vi "element_editor_hydroyse_run.vi"(10 "Break":refnum<vi>) -> ()   [LabVIEW 2019]
uses:
  lib/libSimulationControl/libSimulationControl.lvlib
panel:
  out "spec":path
  # "*******************************************************************\nBiogas Plant Control\n\nAuthor: Paul Zügel\nGCSC-Frankfurt am Main 2020\n\n*******************************************************************"
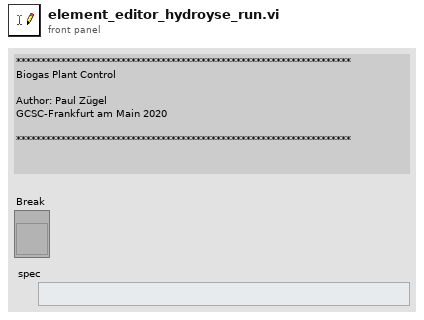
[diagram p1: front panel]
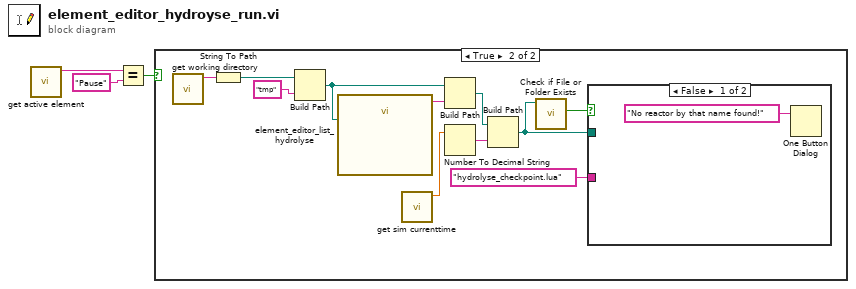
[diagram p0: block diagram]
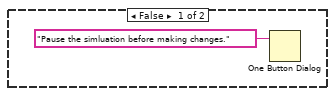
[diagram p2: hidden frame]
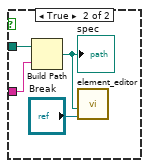
[diagram p3: hidden frame]
diagram:
  n1 = call "get active element.vi"() -> ("active_element"=w3:string)  [unwired: 10 in, 1 out]
  n2 = Equal?(x=w3, y="Pause") -> (x = y?=w1:bool)
  n3 = case shown="True" w1 {
    frame False {
      n4 = One Button Dialog(message="Pause the simluation before making changes.") -> ()  [unwired: 1 in, 1 out]
    }
    frame True {
      n5 = call "get working directory.vi"() -> ("function return"=w10:string)  [unwired: 10 in, 1 out]
      n6 = String To Path(string=w10) -> (path=w11:path)
      n7 = Build Path(base path=w11, name or relative path="tmp") -> (appended path=w5:path)
      n8 = call "element_editor_list_hydrolyse.vi"("path"=w5) -> ("Value"=w6:string)  [unwired: 7 in, 3 out]
      n9 = call "get sim currenttime.vi"() -> ("current_time"=w15:dbl)  [unwired: 10 in, 1 out]
      n10 = Build Path(base path=w5, name or relative path=w6) -> (appended path=w14:path)
      n11 = Number To Decimal String(number=w15) -> (decimal integer string=w13:string)  [unwired: 1 in]
      n12 = Build Path(base path=w14, name or relative path=w13) -> (appended path=w7:path)
      n13 = call <vilib>:"Check if File or Folder Exists.vi"("path"=w7) -> ("file or folder exists?"=w9:bool)  [unwired: 8 in, 2 out]
      n14 = case shown="False" w9 {
        tunnel: "hydrolyse_checkpoint.lua" ("name or relative path") -> [_ w18]
        tunnel: w7 -> [_ w17]
        frame False {
          n15 = One Button Dialog(message="No reactor by that name found!") -> ()  [unwired: 1 in, 1 out]
        }
        frame True {
          n16 = Build Path(base path=w17, name or relative path=w18) -> (appended path=w19:path)
          "spec" <- w19
          n17 = call "element_editor.vi"("Break"="Break", "LUA Specification File"=w19) -> ()  [unwired: 5 in, 1 out]
        }
      }
    }
  }
